vi "Test Method Error Dummy.vi"(8 "error in (no error)":errorcluster, 11 "Setup Error Test Dummy in":refnum<class "Method Error Test Dummy.lvclass">) -> (0 "error out":errorcluster, 3 "Setup Error Test Dummy out":refnum<class "Method Error Test Dummy.lvclass">)   [LabVIEW 2020, in "Method Error Test Dummy.lvclass"]
uses:
  Method Error Test Dummy.lvclass
  LUnit Test Case/LUnit Test Case V2.lvclass/LUnit Test Case V2.ctl
  LUnit Test Case/Private/Append Pass Result.vi
  Method Error Test Dummy.lvclass/Method Error Test Dummy.ctl
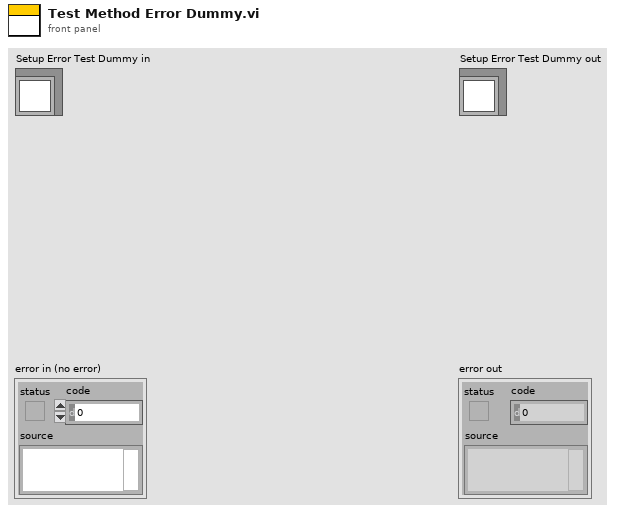
[diagram p1: front panel]
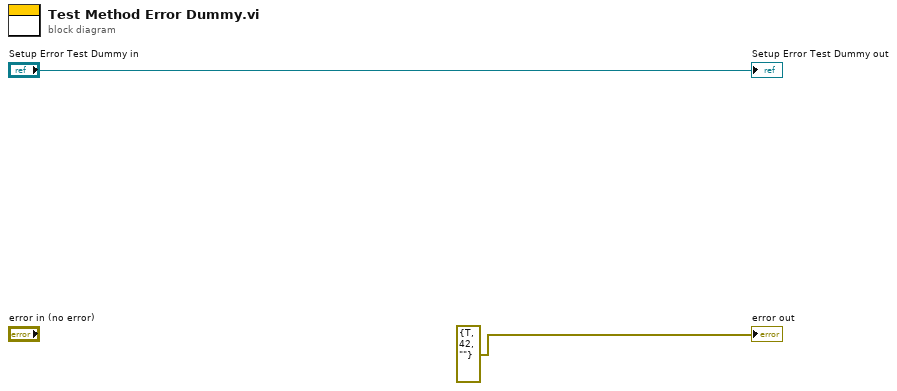
[diagram p0: block diagram]
diagram:
  "error out" <- errorcluster {"status"=TRUE, "code"=42, "source"=""} ("error in (no error)")
  "Setup Error Test Dummy out" <- "Setup Error Test Dummy in"
